vi "SRV_Sensor PARSE_##i(small l).vi"(0 "Return Data":string) -> (3 "Sensor View Indicator Names":T1, 10 "Value":u8)   [LabVIEW 2014]
uses:
  SRV_Sensors Names.ctl
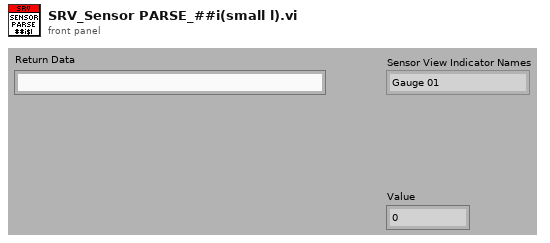
[diagram p1: front panel]
types:
  T1 = typedef "SRV_Sensors Names.ctl" = enum16{"Gauge 01", "Gauge 02", "Gauge 03", "Gauge 04", "Meter 01", "Meter 02", "Meter 03", "Meter 04", "Numeric 01", "Numeric 02", "Numeric 03", "Numeric 04", "Numeric 05", "Numeric 06", "Numeric 07", "Numeric 08", "Boolean 01", "Boolean 02", "Boolean 03", "Boolean 04", "Boolean 05", "Boolean 06", "Boolean 07", "Boolean 08", "Boolean 09", "Boolean 10", "Boolean 11", "Boolean 12", "Boolean 13", "Boolean 14", "Boolean 15", "Boolean 16", "Boolean 17", "Boolean 18", "Boolean 19", "Boolean 20", "Boolean 21", "Boolean 22", "Boolean 23", "Boolean 24", "Boolean 25", "Boolean 26", "Boolean 27", "Boolean 28", "Boolean 29", "Boolean 30", "Boolean 31", "Boolean 32"}
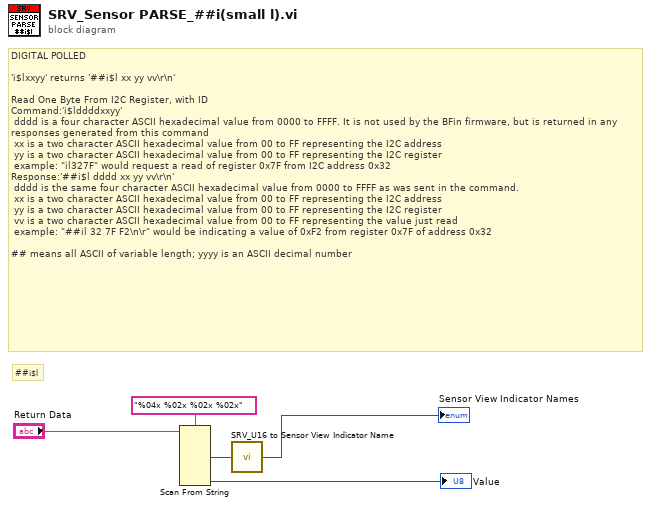
[diagram p0: block diagram]
diagram:
  # "##i$l"
  # "DIGITAL POLLED\n\n'i$lxxyy' returns '##i$l xx yy vv\\r\\n'\n\nRead One Byte From I2C Register, with ID\nCommand:'i$lddddxxyy'\n dddd is a four character ASCII hexadecimal value from 0000 to FFFF. It is not used by the BFin firmware, but is returned in any responses generated from this command\n xx is a two character ASCII hexadecimal value from 00 to FF representing the I2C address\n yy is a two character ASCII hexadecimal value from 00 to FF representing the I2C register\n example: \"il327F\" would request a read of register 0x7F from I2C address 0x32\nResponse:'##i$l dddd xx yy vv\\r\\n'\n dddd is the same four character ASCII hexadecimal value from 0000 to FFFF as was sent in the command.\n xx is a two character ASCII hexadecimal value from 00 to FF representing the I2C address\n yy is a two character ASCII hexadecimal value from 00 to FF representing the I2C register\n vv is a two character ASCII hexadecimal value from 00 to FF representing the value just read\n example: \"##il 32 7F F2\\n\\r\" would be indicating a value of 0xF2 from register 0x7F of address 0x32\n\n## means all ASCII of variable length; yyyy is an ASCII decimal number"
  n1 = Scan From String(format string="%04x %02x %02x %02x", input string="Return Data") -> (output 1=w2:u32, output 4=→"Value":u8)  [unwired: 8 in, 3 out]
  n2 = call "SRV_U16 to Sensor View Indicator Name.vi"("U16"=w2) -> ("Sensor View Indicator Names"=→"Sensor View Indicator Names":T1)  [unwired: 14 in]
